vi "Read Input 2.vi"(8 "error in (no error)":errorcluster, 11 "TECData in":refnum<class "TECData.lvclass">) -> (0 "error out":errorcluster, 2 "Input 2":sgl, 3 "TECData out":refnum<class "TECData.lvclass">)   [LabVIEW 2014, in "TE Cooler.lvlib" / "TECData.lvclass"]
uses:
  TECData.lvclass
  TECData.lvclass/TECData.ctl
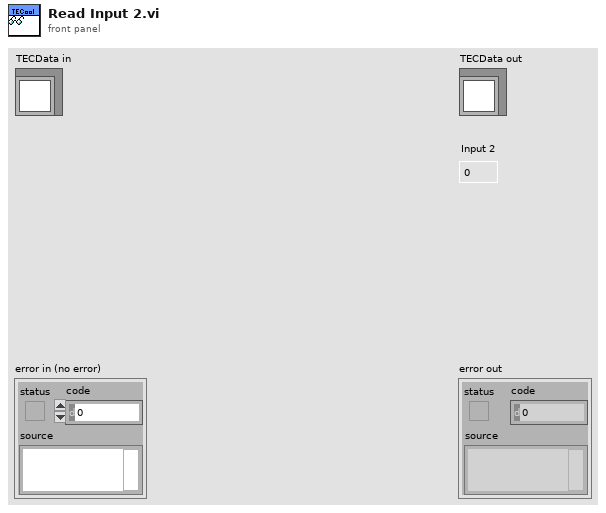
[diagram p1: front panel]
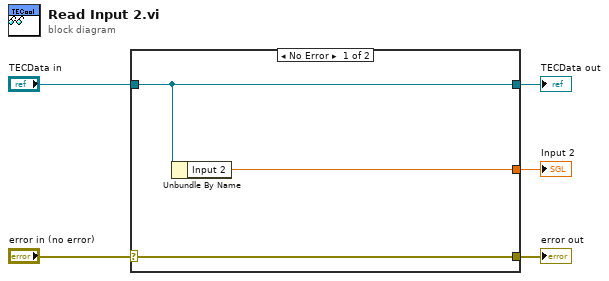
[diagram p0: block diagram]
diagram:
  n1 = case shown="No Error" "error in (no error)" {
    selector: "error in (no error)" -> [w8 w9]
    tunnel: [w8 w9] -> w4
    tunnel: [w7 w10] -> w2
    tunnel: "TECData in" -> [w7 w10]
    tunnel: [w6 _] -> w1
    frame No Error {
      n2 = Unbundle By Name(w7) -> ("Input 2"=w6:sgl)
    }
    frame Error {
    }
  }
  "error out" <- w4
  "TECData out" <- w2
  "Input 2" <- w1
